vi "Test.vi"() -> ()   [LabVIEW 2015, in "Elapsed Time.lvclass"]
uses:
  Elapsed Time.lvclass
panel:
  in  "stop":bool
  out "Elapsed Time (s)":dbl
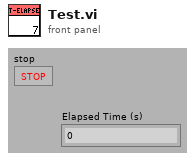
[diagram p1: front panel]
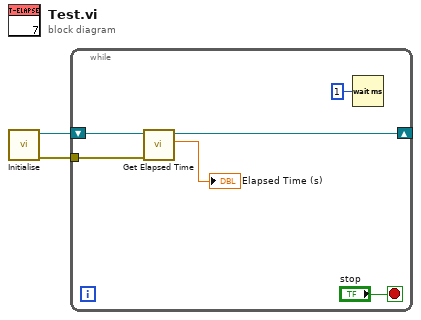
[diagram p0: block diagram]
diagram:
  n1 = call "Initialise.vi"() -> ("error out"=w1:errorcluster, "Elapsed Time out"=w2:refnum<class "Elapsed Time.lvclass">)  [unwired: 1 in, 9 out]
  n2 = while {
    tunnel: w1 -> [w7]
    shift-right: [w4] -> _
    shift-left: w2 -> [w8]
    stop <- "stop" stop-if-true
    n3 = call "Get Elapsed Time.vi"("error in (no error)"=w7, "Elapsed Time.lvclass in"=w8) -> ("Elapsed Time [s]"=→"Elapsed Time (s)":dbl, "Elapsed Time.lvclass out"=w4:refnum<class "Elapsed Time.lvclass">)  [unwired: 8 out]
    n4 = Wait (ms)(milliseconds to wait=u32 1) -> ()  [unwired: 1 out]
  }
